vi "GSP_Manager_CF_driver.vi"(4 "Piezos Setpoints":T1, 5 "error in (no error)":errorcluster, 6 "Target (Move Only)":i32, 7 "Action":T2) -> (0 "error out":errorcluster, 3 "reference out (launch only)":refnum<vi>)   [LabVIEW 2015]
doc: "Provides an interface to the Collimator Focus Manager. See the actions below.\n\nLaunch - launch the manager thread supplying references to the controls that the thread will update.\n\nHome - Home the collimator focus manager\n\nMove - Move the collimator focus to the position supplied by Target\n\nShutdown - Shutdown the collimator focus manager"
uses:
  CF_drivercontrol.ctl
  piezo_setpoint.ctl
  SystemUtil/Command.ctl
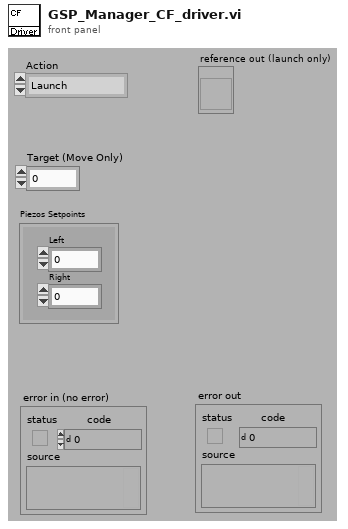
[diagram p1: front panel]
types:
  T1 = typedef "piezo_setpoint.ctl" = cluster{"Left":i32, "Right":i32}
  T2 = typedef "CF_drivercontrol.ctl" = enum16{"Launch", "Move", "Set Piezos", "Flexure On", "Flexure Off", "Home", "Shutdown"}
  T3 = typedef "Command.ctl" = cluster{"Command":string, "Parameter":string}
  T4 = cluster{string, "type string":i16[], "data string":string}
  T5 = cluster{string, "type string":i16[], "data string":string}[]
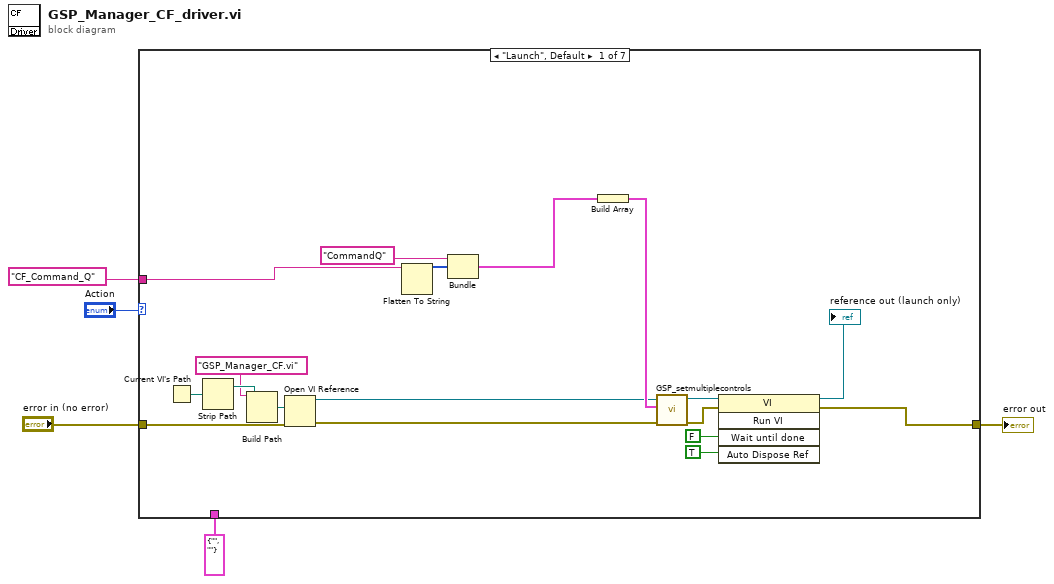
[diagram p0: block diagram]
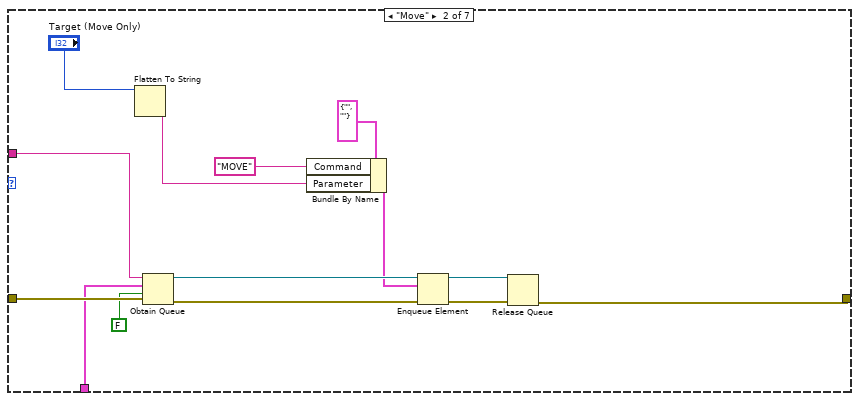
[diagram p2: hidden frame]
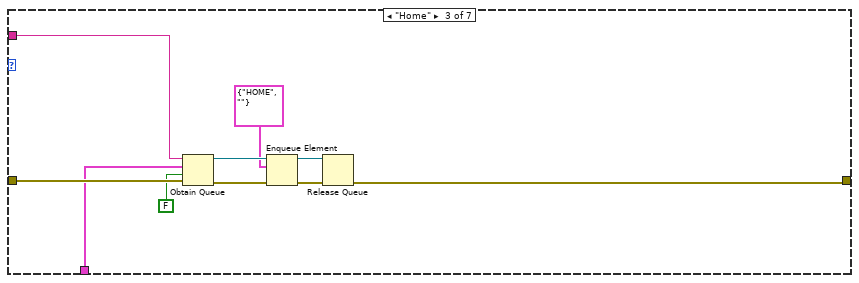
[diagram p3: hidden frame]
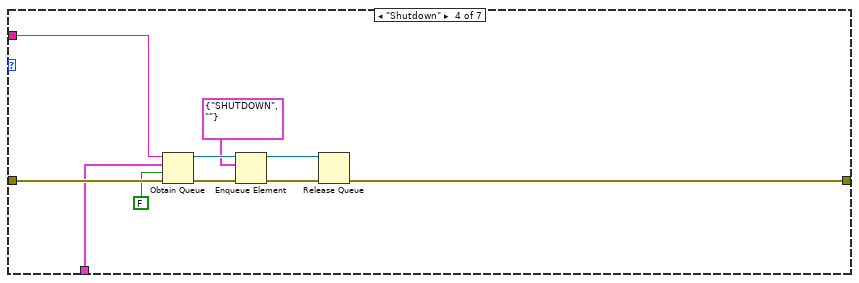
[diagram p4: hidden frame]
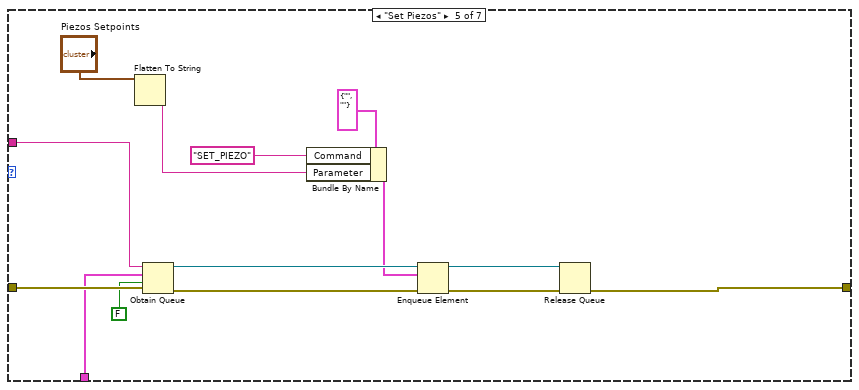
[diagram p5: hidden frame]
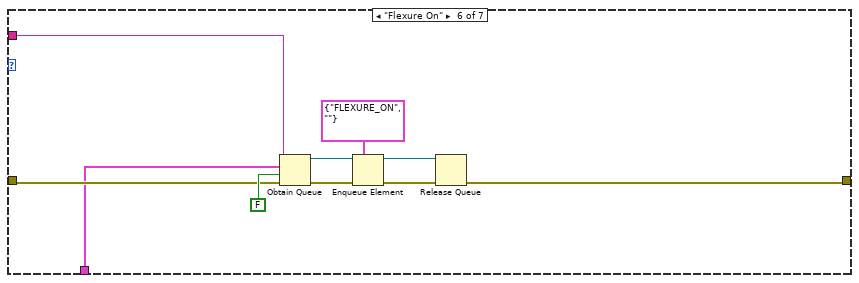
[diagram p6: hidden frame]
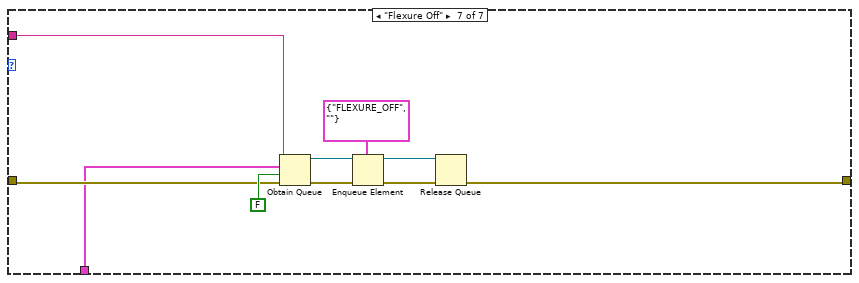
[diagram p7: hidden frame]
diagram:
  n1 = case shown="\"Launch\", Default" "Action" {
    tunnel: "error in (no error)" -> [w20 w38 w46 w58 w72 w76 w86]
    tunnel: [w9 w25 w39 w49 w59 w75 w85] -> w3
    tunnel: "CF_Command_Q" -> [w10 w36 w45 w55 w70 w73 w83]
    tunnel: T3 {"Command"="", "Parameter"=""} ("Command") -> [_ w33 w43 w53 w67 w74 w84]
    frame "Launch", Default {
      n2 = Current VI's Path() -> (path=w14:path)
      n3 = Strip Path(path=w14) -> (stripped path=w12:path)  [unwired: 1 out]
      n4 = Build Path(base path=w12, name or relative path="GSP_Manager_CF.vi" ("vi path")) -> (appended path=w13:path)
      n5 = Open VI Reference(vi path=w13, error in (no error)=w20) -> (vi reference=w8:refnum<vi>, error out=w19:errorcluster)  [unwired: 4 in]
      n6 = Flatten To String(anything=w10) -> (data string=w22:string, type string=w23:i16[])  [unwired: 3 in, 1 out]
      n7 = Bundle("CommandQ", "type string"=w23, "data string"=w22) -> (w7:T4)  [unwired: 1 in]
      n8 = Build Array(w7) -> (w21:T5)
      n9 = call "GSP_setmultiplecontrols.vi"("error in (no error)"=w19, "Control Infos"=w21, "reference"=w8) -> ("error out"=w17:errorcluster, "reference out"=w18:refnum<vi>)  [unwired: 3 in]
      n10 = invoke class="VI" method="Run VI"(reference=w18, error in=w17, "Wait until done"=FALSE, "Auto Dispose Ref"=TRUE) -> (reference out=→"reference out (launch only)":refnum<vi>, error out=w9:errorcluster)  [unwired: 1 in, 3 out]
    }
    frame "Move" {
      n11 = Flatten To String(anything="Target (Move Only)") -> (data string=w28:string)  [unwired: 3 in, 2 out]
      n12 = Obtain Queue(name (unnamed)=w36, element data type=w33, create if not found? (T)=FALSE, error in (no error)=w38) -> (queue out=w35:refnum<queue>, error out=w37:errorcluster)  [unwired: 1 in, 1 out]
      n13 = Bundle By Name(cluster=T3 {"Command"="", "Parameter"=""} ("element"), "Command"="MOVE" ("element"), "Parameter"=w28) -> (w31:T3)
      n14 = Enqueue Element(queue=w35, element=w31, error in (no error)=w37) -> (queue out=w27:refnum<queue>, error out=w26:errorcluster)  [unwired: 1 in, 1 out]
      n15 = Release Queue(queue=w27, error in (no error)=w26) -> (error out=w25:errorcluster)  [unwired: 1 in, 2 out]
    }
    frame "Home" {
      n16 = Obtain Queue(name (unnamed)=w45, element data type=w43, create if not found? (T)=FALSE, error in (no error)=w46) -> (queue out=w47:refnum<queue>, error out=w48:errorcluster)  [unwired: 1 in, 1 out]
      n17 = Enqueue Element(queue=w47, element=T3 {"Command"="HOME", "Parameter"=""}, error in (no error)=w48) -> (queue out=w41:refnum<queue>, error out=w40:errorcluster)  [unwired: 1 in, 1 out]
      n18 = Release Queue(queue=w41, error in (no error)=w40) -> (error out=w39:errorcluster)  [unwired: 1 in, 2 out]
    }
    frame "Shutdown" {
      n19 = Obtain Queue(name (unnamed)=w55, element data type=w53, create if not found? (T)=FALSE, error in (no error)=w58) -> (queue out=w56:refnum<queue>, error out=w57:errorcluster)  [unwired: 1 in, 1 out]
      n20 = Enqueue Element(queue=w56, element=T3 {"Command"="SHUTDOWN", "Parameter"=""}, error in (no error)=w57) -> (queue out=w51:refnum<queue>, error out=w50:errorcluster)  [unwired: 1 in, 1 out]
      n21 = Release Queue(queue=w51, error in (no error)=w50) -> (error out=w49:errorcluster)  [unwired: 1 in, 2 out]
    }
    frame "Set Piezos" {
      n22 = Flatten To String(anything="Piezos Setpoints") -> (data string=w63:string)  [unwired: 3 in, 2 out]
      n23 = Obtain Queue(name (unnamed)=w70, element data type=w67, create if not found? (T)=FALSE, error in (no error)=w72) -> (queue out=w69:refnum<queue>, error out=w71:errorcluster)  [unwired: 1 in, 1 out]
      n24 = Bundle By Name(cluster=T3 {"Command"="", "Parameter"=""} ("element"), "Command"="SET_PIEZO" ("element"), "Parameter"=w63) -> (w65:T3)
      n25 = Enqueue Element(queue=w69, element=w65, error in (no error)=w71) -> (queue out=w61:refnum<queue>, error out=w60:errorcluster)  [unwired: 1 in, 1 out]
      n26 = Release Queue(queue=w61, error in (no error)=w60) -> (error out=w59:errorcluster)  [unwired: 1 in, 2 out]
    }
    frame "Flexure On" {
      n27 = Obtain Queue(name (unnamed)=w73, element data type=w74, create if not found? (T)=FALSE, error in (no error)=w76) -> (queue out=w81:refnum<queue>, error out=w82:errorcluster)  [unwired: 1 in, 1 out]
      n28 = Enqueue Element(queue=w81, element=T3 {"Command"="FLEXURE_ON", "Parameter"=""}, error in (no error)=w82) -> (queue out=w78:refnum<queue>, error out=w77:errorcluster)  [unwired: 1 in, 1 out]
      n29 = Release Queue(queue=w78, error in (no error)=w77) -> (error out=w75:errorcluster)  [unwired: 1 in, 2 out]
    }
    frame "Flexure Off" {
      n30 = Obtain Queue(name (unnamed)=w83, element data type=w84, create if not found? (T)=FALSE, error in (no error)=w86) -> (queue out=w91:refnum<queue>, error out=w92:errorcluster)  [unwired: 1 in, 1 out]
      n31 = Enqueue Element(queue=w91, element=T3 {"Command"="FLEXURE_OFF", "Parameter"=""}, error in (no error)=w92) -> (queue out=w88:refnum<queue>, error out=w87:errorcluster)  [unwired: 1 in, 1 out]
      n32 = Release Queue(queue=w88, error in (no error)=w87) -> (error out=w85:errorcluster)  [unwired: 1 in, 2 out]
    }
  }
  "error out" <- w3
